vi "idn_action.vi"(0 "NInstrSim":refnum<class "NInstrSim.lvclass">, 5 "error in (no error)":errorcluster) -> (12 "resourceString":string, 13 "additionalInfo":string, 14 "dup NInstrSim":refnum<class "NInstrSim.lvclass">, 15 "driverRevision":string="unknown", 16 "firmwareRevision":string="unknown", 17 "vendor":string="unknown", 18 "model":string="unknown", 19 "error out":errorcluster)   [LabVIEW 2009, in "HB_Device_Examples.lvlib" / "NInstrSim.lvclass"]
doc: "This VI queries the current instrument firmware revision and instrument driver revision.\n\nFor detailed driver information including modification history, refer to the Readme file.\n\n<b>Hint:</b> This is a dynamic dispatch VI to be implemented by child classes."
uses:
  NInstrSim.lvclass
  lib.lib/HGF_LVC/HGF_DeviceBaseClasses/HGF_VISADevice/HGF_VISADevice.lvclass
  non_GPL/instr.lib/NI Instrument Simulator/NI Instrument Simulator.lvlib
  lib.lib/HGF_LVC/HGF_DeviceBaseClasses/HGF_DeviceBase/HGF_DeviceBase.lvclass
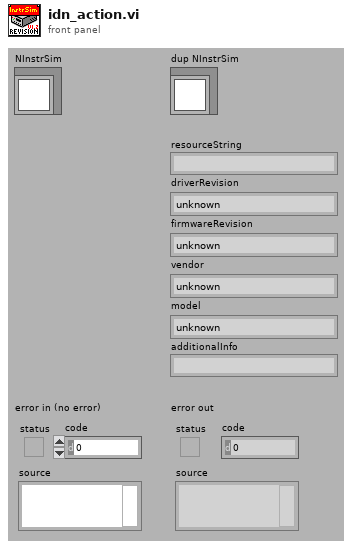
[diagram p1: front panel]
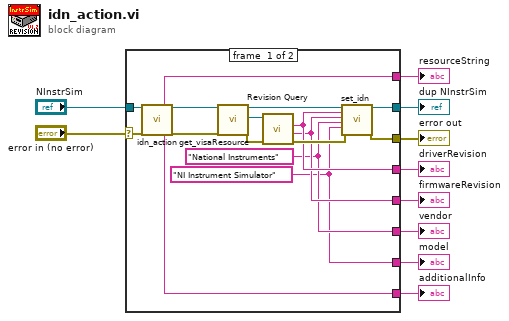
[diagram p0: block diagram]
diagram:
  n1 = case shown="No Error" "error in (no error)" {
    selector: "error in (no error)" -> [w15 w27]
    tunnel: "NInstrSim" -> [w16 w28]
    tunnel: [w24 w28] -> w9
    tunnel: [w21 w27] -> w8
    tunnel: [w20 _] -> w6
    tunnel: [w19 _] -> w5
    tunnel: [w18 _] -> w4
    tunnel: [w17 _] -> w3
    tunnel: [w12 _] -> w2
    tunnel: [w11 _] -> w1
    frame #0 {
      w17 = "NI Instrument Simulator" ("model")
      w18 = "National Instruments" ("vendor")
      n2 = call-parent "idn_action.vi"("HGF_VISADevice"=w16, "error in (no error)"=w15) -> ("resourceString"=w12:string, "additionalInfo"=w11:string, "dup HGF_VISADevice"=w13:refnum<class "NInstrSim.lvclass">, "error out"=w14:errorcluster)  [unwired: 14 out]
      n3 = call "get_visaResource.vi"("HGF_VISADevice"=w13, "error in (no error)"=w14) -> ("dup HGF_VISADevice"=w25:refnum<class "NInstrSim.lvclass">, "VISA Resource Name"=w26:refnum<visa-resource-name>, "error out"=w23:errorcluster)  [unwired: 15 out]
      n4 = call "Revision Query.vi"("error in (no error)"=w23, "VISA resource name"=w26) -> ("error out"=w22:errorcluster, "Instrument Firmware Revision"=w19:string, "Instrument Driver Revision"=w20:string)  [unwired: 7 out]
      n5 = call "set_idn.vi"("HGF_DeviceBase"=w25, "driverRevision"=w20, "firmwareRevision"=w19, "vendor"=w18, "model"=w17, "error in (no error)"=w22) -> ("dup HGF_DeviceBase"=w24:refnum<class "NInstrSim.lvclass">, "error out"=w21:errorcluster)  [unwired: 12 out]
    }
    frame #1 {
    }
  }
  "error out" <- w8
  "dup NInstrSim" <- w9
  "model" <- w3
  "firmwareRevision" <- w5
  "driverRevision" <- w6
  "vendor" <- w4
  "resourceString" <- w2
  "additionalInfo" <- w1
